vi "Service Request Enable Query.vi"(0 "VISA resource name":refnum<visa-resource-name>, 11 "error in (no error)":errorcluster) -> (4 "VISA resource name out":refnum<visa-resource-name>, 6 "Service Request Enable":T1, 15 "error out":errorcluster)   [LabVIEW 2018, in "XP Power PLS600.lvlib"]
doc: "Queries the Service Request enable register. Returns the decimal value of binary-weighted sum of bits.\n\nThe Service Request Event Register consists of the following 8 bits.\n\nBIT 0: Reserved\nBIT 1: Reserved\nBIT 2: Error in Queue\nBIT 3: QUES = Questionable Status Summary\nBIT 4: MAV = Message Available\nBIT 5: ESB = Event Status Byte Summary\nBIT 6: RQS = Request for Service\nBIT 7: OPER = Operation Event Summary"
uses:
  XP Power PLS600.lvlib
panel:
  # "BIT 0: Reserved\nBIT 1: Reserved\nBIT 2: Error in Queue\nBIT 3: QUES = Questionable Status Summary\nBIT 4: MAV = Message Available\nBIT 5: ESB = Event Status Byte Summary\nBIT 6: RQS = Request for Service\nBIT 7: OPER = Operation Event Summary"
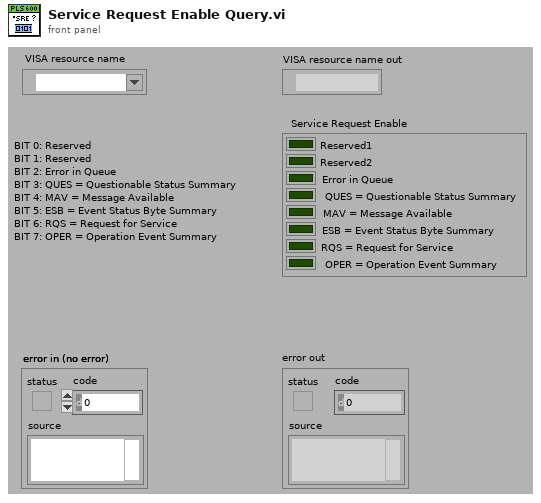
[diagram p1: front panel]
types:
  T1 = cluster{"Reserved1":bool, "Reserved2":bool, "Error in Queue":bool, "QUES = Questionable Status Summary":bool, "MAV = Message Available":bool, "ESB = Event Status Byte Summary":bool, "RQS = Request for Service":bool, "OPER = Operation Event Summary":bool}
  T2 = cluster{"Boolean array[0]":bool, "Boolean array[1]":bool, "Boolean array[2]":bool, "Boolean array[3]":bool, "Boolean array[4]":bool, "Boolean array[5]":bool, "Boolean array[6]":bool, "Boolean array[7]":bool}
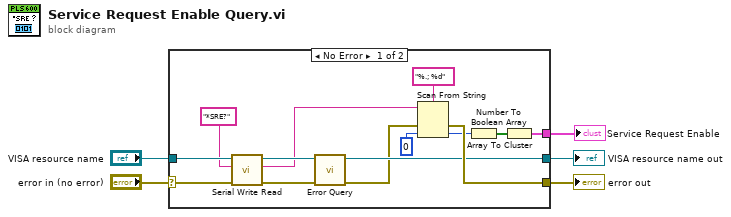
[diagram p0: block diagram]
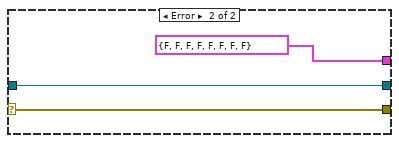
[diagram p2: hidden frame]
diagram:
  n1 = case shown="No Error" "error in (no error)" {
    selector: "error in (no error)" -> [w10 w22]
    tunnel: [w16 T2 {"Boolean array[0]"=FALSE, "Boolean array[1]"=FALSE, "Boolean array[2]"=FALSE, "Boolean array[3]"=FALSE, "Boolean array[4]"=FALSE, "Boolean array[5]"=FALSE, "Boolean array[6]"=FALSE, "Boolean array[7]"=FALSE} ("Boolean array")] -> w1
    tunnel: "VISA resource name" -> [w11 w21]
    tunnel: [w8 w21] -> w4
    tunnel: [w15 w22] -> w3
    frame No Error {
      n2 = call "Serial Write Read.vi"("error in (no error)"=w10, "Write Buffer"="*SRE?" ("Command to Send (empty)"), "VISA resource name"=w11) -> ("error out"=w13:errorcluster, "Read Buffer"=w6:string, "VISA resource name out"=w12:refnum<visa-resource-name>)  [unwired: 6 in]
      n3 = call "Error Query.vi"("error in (no error)"=w13, "VISA resource name"=w12) -> ("error out"=w7:errorcluster, "VISA resource name out"=w8:refnum<visa-resource-name>)  [unwired: 6 in, 2 out]
      n4 = Scan From String(format string="%.; %d" ("Format String"), input string=w6, error in=w7, default 1=u8 0 ("default value 1")) -> (error out=w15:errorcluster, output 1=w14:u8)  [unwired: 1 in, 2 out]
      n5 = Number To Boolean Array(number=w14) -> (Boolean array=w17:bool[])
      n6 = Array To Cluster(array=w17) -> (cluster=w16:T2)
    }
    frame Error {
    }
  }
  "error out" <- w3
  "VISA resource name out" <- w4
  "Service Request Enable" <- w1
